vi "CorrectResponse.vi"(8 "error in (no error)":errorcluster, 11 "TrialBasedExperiment in":refnum<class "TrialBasedExperiment.lvclass">) -> (0 "error out":errorcluster, 3 "TrialBasedExperiment out":refnum<class "TrialBasedExperiment.lvclass">)   [LabVIEW 2014, in "AcquisitionCoreObjects.lvlib" / "TrialBasedExperiment.lvclass"]
uses:
  TrialBasedExperiment.lvclass
  TrialBasedExperiment.lvclass/TrialBasedExperiment.ctl
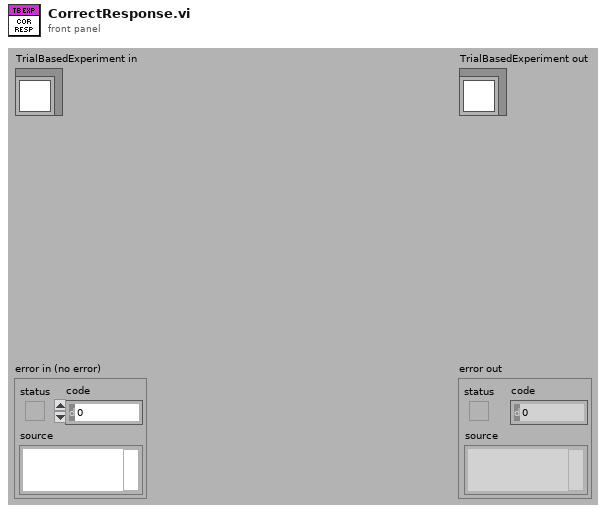
[diagram p1: front panel]
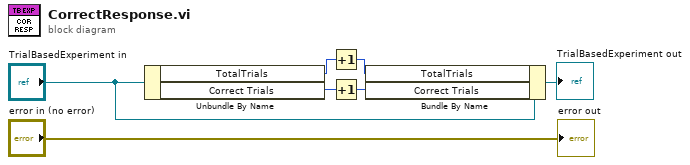
[diagram p0: block diagram]
diagram:
  n1 = Unbundle By Name("TrialBasedExperiment in") -> ("TotalTrials"=w4:u32, "Correct Trials"=w7:u32)
  n2 = Increment(x=w4) -> (x+1=w3:u32)
  n3 = Increment(x=w7) -> (x+1=w6:u32)
  n4 = Bundle By Name(cluster="TrialBasedExperiment in", "TotalTrials"=w3, "Correct Trials"=w6) -> (→"TrialBasedExperiment out":refnum<class "TrialBasedExperiment.lvclass">)
  "error out" <- "error in (no error)"
